vi "Simple Dialog.vi"() -> ()   [LabVIEW 2017]
doc: "This is a simple dialog that demonstrates the Panel VI defining what type of panel class to use.\n----\nCopyright: MGI 2016\nAuthor: Derek Trepanier"
uses:
  panel-manager/Source/Panel/Window/Dialog/Dialog.lvclass
  panel-manager/Source/Panel/Panel.lvclass
  D:/test/LabView_PanelManager/panel-manager/Source/Panel/Panel.lvclass
panel:
  in  "OK":bool
  # "Example Dialog"
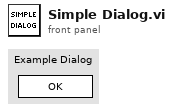
[diagram p1: front panel]
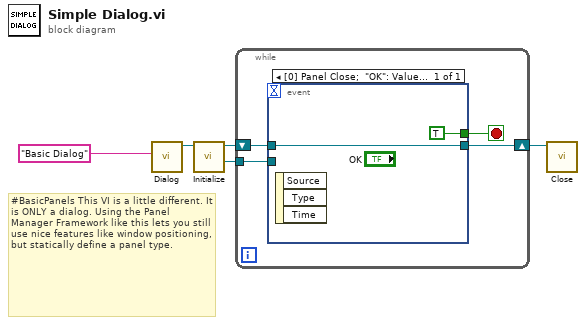
[diagram p0: block diagram]
diagram:
  # "#BasicPanels This VI is a little different. It is ONLY a dialog. Using the Panel Manager Framework like this lets you still use nice features like window positioning, but statically define a panel type."
  n1 = call "Dialog.vi"("Default Title"="Basic Dialog" ("Title")) -> ("Dialog out"=w5:refnum<class "Dialog.lvclass">)  [unwired: 9 in, 1 out]
  n2 = call "Initialize.vi"("Panel In"=w5) -> ("My Helper out"=w1:refnum<class "Panel Helper.lvclass">, "Panel Out"=w3:refnum<class "Dialog.lvclass">)  [unwired: 8 in, 1 out]
  n3 = while {
    shift-right: [w9] -> w4
    shift-left: w3 -> [w8]
    tunnel: w1 -> [w6]
    stop <- w7 stop-if-true
    n4 = event shown="[0] Panel Close;  \"OK\": Value Change" {
      selector: _ -> [_]
      dyn-events: _ -> [_]
      timeout: _ -> [_]
      tunnel: [w11] -> w9
      tunnel: w8 -> [w11]
      tunnel: [TRUE] -> w7
      tunnel: w6 -> [_]
      event Panel Close; "OK": Value Change {
        n5 = event-data() -> ()  [unwired: 1 in, 3 out]
      }
    }
  }
  n6 = call-dynamic "Close.vi"("Dialog in"=w4) -> ()  [unwired: 10 in, 1 out]
